vi "Excit_Process_Signal.vi"(4 "Excit Form":T1, 5 "Factor":dbl=0.8 format="%#_13g", 6 "Duration (µs)":dbl=800.0, 7 "Sampling Frequency (MHz)":dbl=20.0, 8 "End Frequency (kHz)":dbl=250.0, 9 "Start Frequency (kHz)":dbl=250.0, 10 "Amplitude (%)":dbl=100.0) -> (0 "FFT Excitation":dbl[](array[numeric]), 1 "X Freq":dbl[](array[numeric]), 2 "Signal Excitation":dbl[](array[numeric]), 3 "X Time":dbl[](array[numeric]))   [LabVIEW 2018]
doc: "From a start and end value, generates an adiabatic waveform signal of 2000 values (double).\nWrites this waveform into a binary file, in a big-endian format.\nDisplays the written data and the FFT of the signal.\nDefault Path for the generated file is D:\\PIRENEA\\EXCIT_WFMS\n\nAvailable Waveforms : Sinus, Swift, Chirp, Ramp (Up or Down), DoubleRamp (Up-Down or Down-Up)"
uses:
  controls/EXCIT_Form_Selector.ctl
  <vilib>/Analysis/2dsp.llb/Inverse Complex FFT.vi
  <vilib>/Analysis/NI_AALPro.lvlib
panel:
  out "error out":errorcluster caption="sortie d'erreur"
  in  "error in (no error)":errorcluster
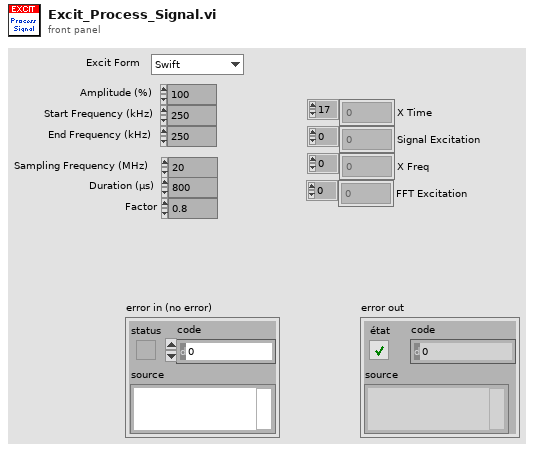
[diagram p1: front panel]
types:
  T1 = typedef "EXCIT_Form_Selector.ctl" = enum16{"Swift", "TwoSwift", "Chirp", "Sinus", "Ramp"}
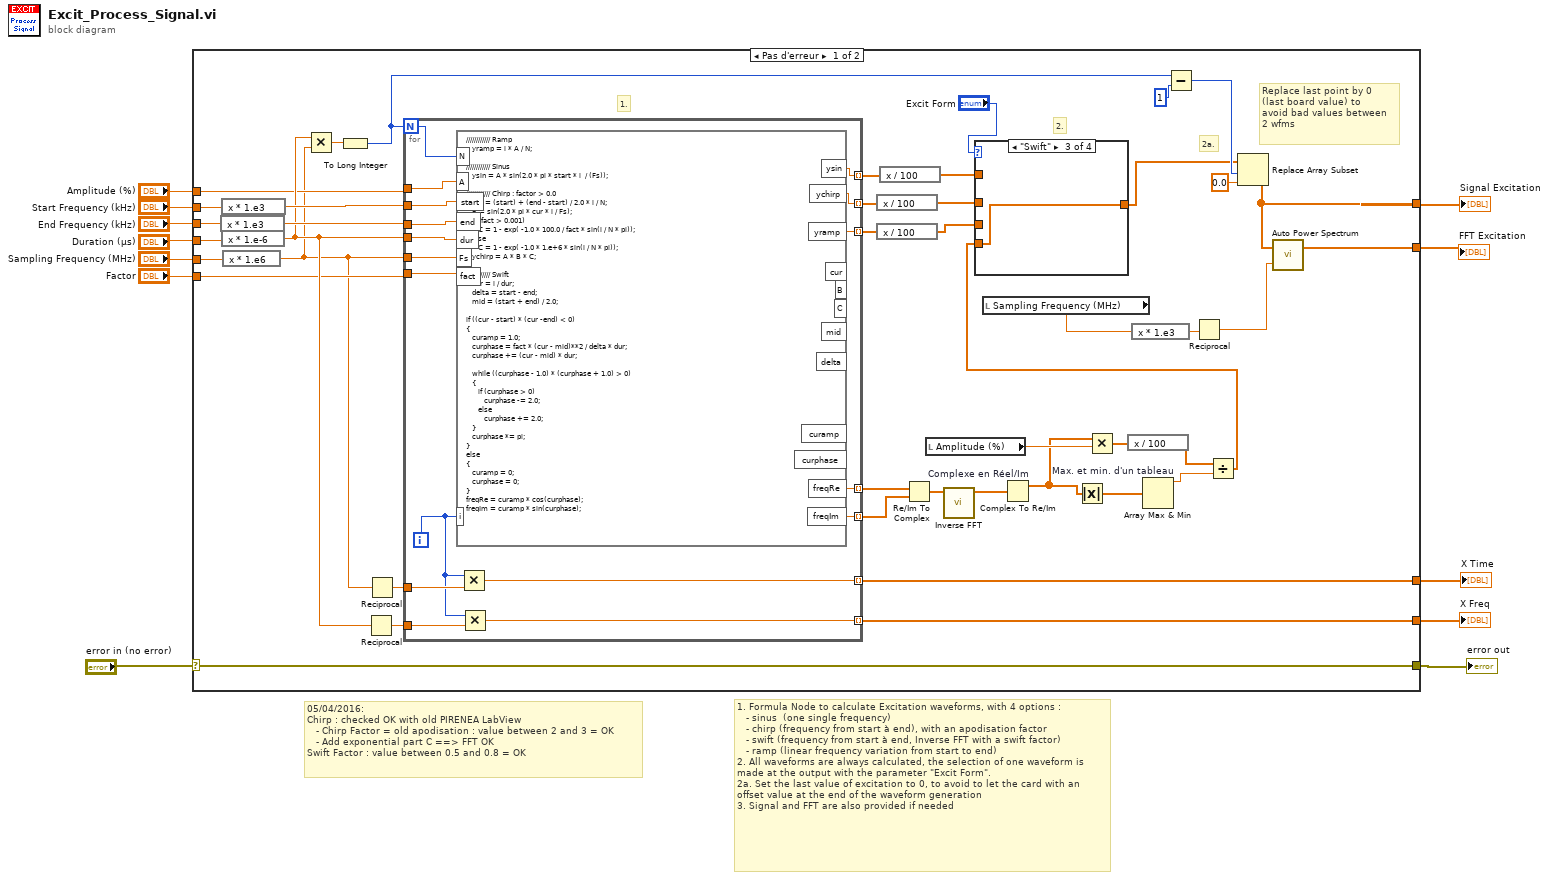
[diagram p0: block diagram]
diagram:
  # "05/04/2016:\nChirp : checked OK with old PIRENEA LabView\n   - Chirp Factor = old apodisation : value between 2 and 3 = OK\n   - Add exponential part C ==> FFT OK\nSwift Factor : value between 0.5 and 0.8 = OK"
  # "1. Formula Node to calculate Excitation waveforms, with 4 options :\n   - sinus  (one single frequency)\n   - chirp (frequency from start à end), with an apodisation factor\n   - swift (frequency from start à end, Inverse FFT with a swift factor)\n   - ramp (linear frequency variation from start to end)\n2. All waveforms are always calculated, the selection of one waveform is made at the output with the parameter \"Excit Form\".\n2a. Set the last value of excitation to 0, to avoid to let the card with an offset value at the end of the waveform generation\n3. Signal and FFT are also provided if needed"
  n1 = case shown="Pas d'erreur" "error in (no error)" {
    selector: "error in (no error)" -> [w13 w78]
    tunnel: [w38 _] -> w12
    tunnel: [w34 _] -> w11
    tunnel: "Amplitude (%)" -> [w31 _]
    tunnel: "Start Frequency (kHz)" -> [w30 _]
    tunnel: "End Frequency (kHz)" -> [w29 _]
    tunnel: "Duration (µs)" -> [w28 _]
    tunnel: "Sampling Frequency (MHz)" -> [w27 _]
    tunnel: "Factor" -> [w26 _]
    tunnel: [w24 _] -> w4
    tunnel: [w18 _] -> w3
    tunnel: [w13 w78] -> w1
    frame No Error {
      # "Replace last point by 0\n(last board value) to\navoid bad values between\n2 wfms"
      # "2a."
      # "2."
      # "1."
      n2 = expression code="x * 1.e3"(w29) -> (w55:dbl)
      n3 = expression code="x * 1.e3"(w30) -> (w56:dbl)
      n4 = expression code="x * 1.e-6"(w28) -> (w36:dbl)
      n5 = expression code="x * 1.e6"(w27) -> (w16:dbl)
      n6 = Multiply(x=w36, y=w16) -> (x*y=w48:dbl)
      n7 = To Long Integer(number=w48) -> (32bit integer=w21:i32)
      n8 = Reciprocal(x=w36) -> (1/x=w35:dbl)
      n9 = Reciprocal(x=w16) -> (1/x=w37:dbl)
      n10 = for {
        N: w21 -> [w77]
        tunnel: [w76] -> w45 mode=indexing
        tunnel: w55 -> [w72]
        tunnel: [w75] -> w47 mode=indexing
        tunnel: w56 -> [w73]
        tunnel: w31 -> [w74]
        tunnel: w36 -> [w70]
        tunnel: w16 -> [w71]
        tunnel: [w69] -> w52 mode=indexing
        tunnel: [w68] -> w51 mode=indexing
        tunnel: w26 -> [w67]
        tunnel: [w66] -> w41 mode=indexing
        tunnel: w37 -> [w65]
        tunnel: [w64] -> w38 mode=indexing
        tunnel: w35 -> [w62]
        tunnel: [w61] -> w34 mode=indexing
        i -> [w63]
        n11 = formula code="//////////// Ramp\n   yramp = i * A / N;\n\n//////////// Sinus\n   ysin = A * sin(2.0 * pi * start * i  / (Fs));\n\n//////////// Chirp : factor > 0.0\n   cur = (start) + (end - start) / 2.0 * i / N;\n   B = sin(2.0 * pi * cur * i / Fs);\n   if (fact > 0.001)\n      C = 1 - exp( -1.0 * 100.0 / fact * sin(i / N * pi));\n   else\n      C = 1 - exp( -1.0 * 1.e+6 * sin(i / N * pi));\n   ychirp = A * B * C;\n   \n//////////// Swift\n   cur = i / dur;\n   delta = start - end;\n   mid = (start + end) / 2.0;\n\nif ((cur - start) * (cur -end) < 0)\n{\n   curamp = 1.0;\n   curphase = fact * (cur - mid)**2 / delta * dur;\n   curphase += (cur - mid) * dur;\n\n   while ((curphase - 1.0) * (curphase + 1.0) > 0)\n   {\n      if (curphase > 0)\n         curphase -= 2.0;\n      else\n         curphase += 2.0;\n   }\n   curphase *= pi;\n}\nelse\n{\n   curamp = 0;\n   curphase = 0;\n}\nfreqRe = curamp * cos(curphase);\nfreqIm = curamp * sin(curphase);"("A"=w74, "start"=w73, "i"=w63, "N"=w77, "end"=w72, "Fs"=w71, "dur"=w70, "fact"=w67) -> ("ychirp"=w76:dbl, "ysin"=w75:dbl, "freqRe"=w69:dbl, "freqIm"=w68:dbl, "yramp"=w66:dbl)  [unwired: 7 out]
        n12 = Multiply(x=w63, y=w65) -> (x*y=w64:dbl)
        n13 = Multiply(x=w63, y=w62) -> (x*y=w61:dbl)
      }
      n14 = expression code="x / 100"(w45) -> (w44:dbl[])
      n15 = expression code="x / 100"(w41) -> (w40:dbl[])
      n16 = expression code="x / 100"(w47) -> (w46:dbl[])
      n17 = Re/Im To Complex(1:w51, 2:w52) -> (0:w50:cdb[])
      n18 = local read "Amplitude (%)"() -> (w39:dbl)
      n19 = call-poly <vilib>:"Inverse FFT.vi"("FFT {X}"=w50) -> ("X"=w53:cdb[])  [unwired: 9 in, 1 out]
      n20 = local read "Sampling Frequency (MHz)"() -> (w17:dbl)
      n21 = Complex To Re/Im "Complexe en Réel/Im"(x + iy=w53) -> (x=w15:dbl[])  [unwired: 1 out]
      n22 = Absolute Value(x=w15) -> (abs(x)=w14:dbl[])
      n23 = Multiply(x=w15, y=w39) -> (x*y=w43:dbl[])
      n24 = expression code="x / 100"(w43) -> (w42:dbl[])
      n25 = expression code="x * 1.e3"(w17) -> (w32:dbl)
      n26 = Array Max & Min "Max. et min. d'un tableau"(array=w14) -> (max value=w54:dbl)  [unwired: 3 out]
      n27 = Subtract(x=w21, y=1) -> (x-y=w20:i32)
      n28 = Reciprocal(x=w32) -> (1/x=w33:dbl)
      n29 = Divide(x=w42, y=w54) -> (x/y=w49:dbl[])
      n30 = case shown="\"Swift\"" "Excit Form" {
        tunnel: [w57 w58 w59 w60] -> w19
        tunnel: w49 -> [_ _ w59 _]
        tunnel: w46 -> [w57 _ _ _]
        tunnel: w44 -> [_ w58 _ _]
        tunnel: w40 -> [_ _ _ w60]
        frame "Sinus", Default {
        }
        frame "Chirp" {
        }
        frame "Swift" {
        }
        frame "Ramp" {
        }
      }
      n31 = Replace Array Subset(array=w19, new element=0.0 ("nouvel élément/sous-tableau"), index=w20) -> (w18:dbl[])
      n32 = call <vilib>:"Auto Power Spectrum.vi"("dt"=w33, "Signal (V)"=w18) -> ("Power Spectrum (V^2 rms)"=w24:dbl[])  [unwired: 1 out]
    }
    frame Error {
    }
  }
  "X Time" <- w12
  "X Freq" <- w11
  "Signal Excitation" <- w3
  "FFT Excitation" <- w4
  "error out" <- w1
